vi "Search for Added and Removed Items - String Array.vi"(8 "Model":string[](array[string]), 11 "SysDef":string[](array[string])) -> (1 "Model Items Removed":string[](array[string]), 3 "Model Items Added":string[](array[string]))   [LabVIEW 2016]
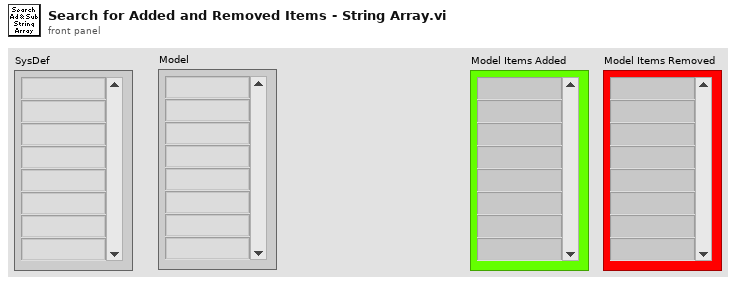
[diagram p1: front panel]
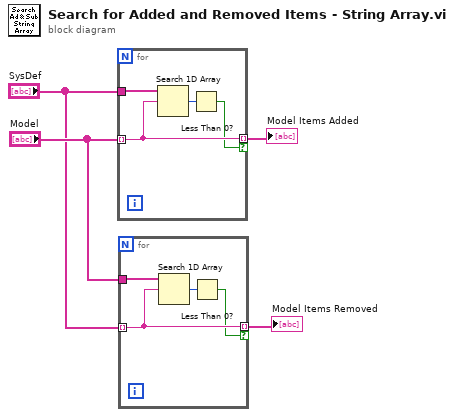
[diagram p0: block diagram]
diagram:
  n1 = for {
    tunnel: "SysDef" -> [w8]
    tunnel: "Model" -> [w6] mode=indexing
    tunnel: [w6] -> w4 mode=indexing if=w5
    n2 = Search 1D Array(1D array=w8, element=w6) -> (index of element=w7:i32)  [unwired: 1 in]
    n3 = Less Than 0?(x=w7) -> (x < 0?=w5:bool)
  }
  "Model Items Added" <- w4
  n4 = for {
    tunnel: "Model" -> [w12]
    tunnel: "SysDef" -> [w10] mode=indexing
    tunnel: [w10] -> w1 mode=indexing if=w9
    n5 = Search 1D Array(1D array=w12, element=w10) -> (index of element=w11:i32)  [unwired: 1 in]
    n6 = Less Than 0?(x=w11) -> (x < 0?=w9:bool)
  }
  "Model Items Removed" <- w1
